vi "Read TemplatesFolder Key.vi"(8 "Error In":errorcluster) -> (0 "Error Out":errorcluster, 3 "Templates Folder Path":path)   [LabVIEW 2022 SP3]
doc: "This VI reads the path of the folder that stores the template VIs and CTLs from the \"TemplatesFolder\" value of the Windows Registry Key HKEY_CURRENT_USER\\Software\\NewViFromTemplate .\n\nIf the HKEY_CURRENT_USER\\Software\\NewViFromTemplate key doesn't exist, this VI creates it, and the \"TemplatesFolder\" value.\n\nIf the HKEY_CURRENT_USER\\Software\\NewViFromTemplate key exists, but the \"TemplatesFolder\" value doesn't, this VI creates the \"TemplatesFolder\" value.\n\nPetru, 07 November 2022"
uses:
  <vilib>/registry/registry.llb/Read Registry Value Simple STR.vi
  <vilib>/registry/registry.llb/Write Registry Value Simple STR.vi
panel:
  # "Development\nControls or indicators that are useful for development or testing, but which are not outputs of the VI."
  # "Input\nInputs to the VI"
  # "Output\nOutputs of the VI"
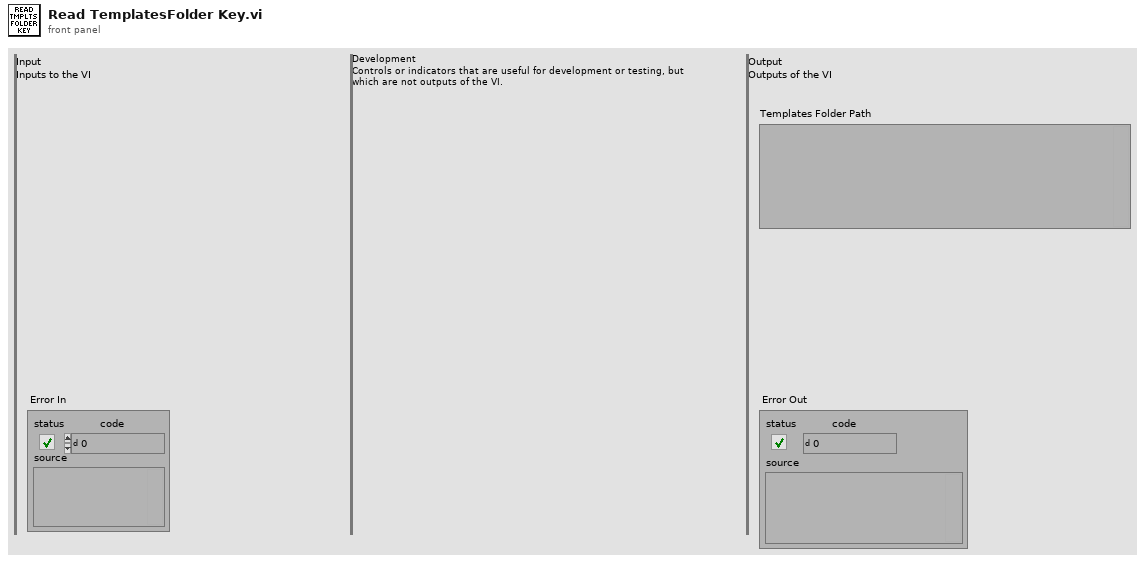
[diagram p1: front panel]
types:
  T1 = typedef "Registry RtKey.ctl" = enum32{"HKEY_CLASSES_ROOT", "HKEY_CURRENT_USER", "HKEY_LOCAL_MACHINE", "HKEY_USERS", "HKEY_PERFORMANCE_DATA", "HKEY_CURRENT_CONFIG", "HKEY_DYN_DATA"}
  T2 = typedef "Registry refnum.ctl" = refnum<k1>
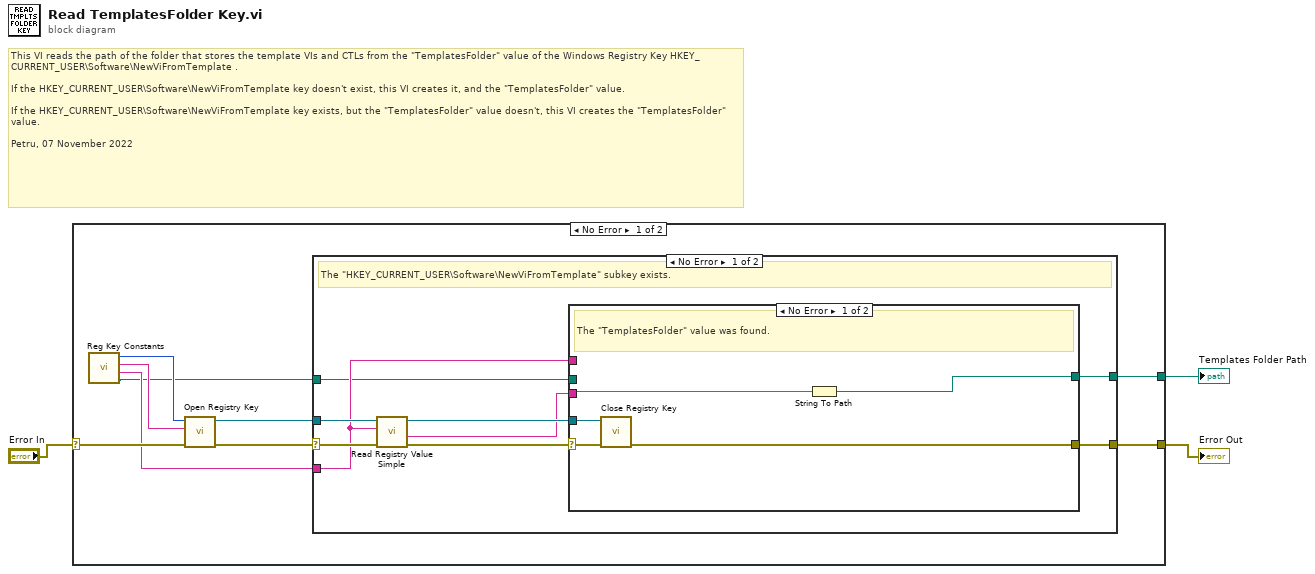
[diagram p0: block diagram]
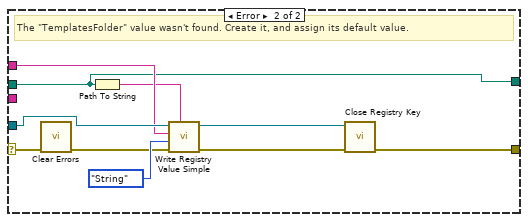
[diagram p2: hidden frame]
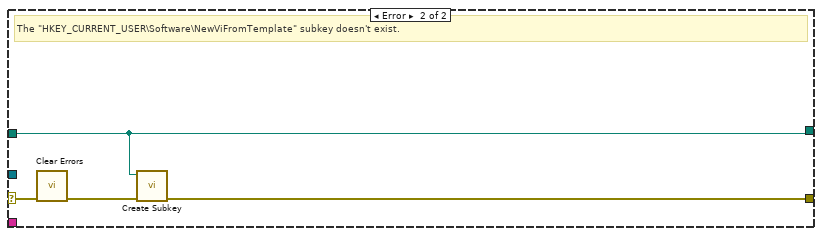
[diagram p3: hidden frame]
diagram:
  # "This VI reads the path of the folder that stores the template VIs and CTLs from the \"TemplatesFolder\" value of the Windows Registry Key HKEY_CURRENT_USER\\Software\\NewViFromTemplate .\n\nIf the HKEY_CURRENT_USER\\Software\\NewViFromTemplate key doesn't exist, this VI creates it, and the \"TemplatesFolder\" value.\n\nIf the HKEY_CURRENT_USER\\Software\\NewViFromTemplate key exists, but the \"TemplatesFolder\" value doesn't, this VI creates the \"TemplatesFolder\" value.\n\nPetru, 07 November 2022"
  n1 = case shown="No Error" "Error In" {
    selector: "Error In" -> [w12 w41]
    tunnel: [w10 w41] -> w2
    tunnel: [w8 _] -> w1
    frame No Error {
      n2 = call "Reg Key Constants.vi"() -> ("Default Templates Folder"=w4:path, "Name of TemplatesFolder Value"=w5:string, "Subkey Path"=w6:string, "Root Key"=w7:T1)  [unwired: 3 in, 1 out]
      n3 = call <vilib>:"Open Registry Key.vi"("error in (no error)"=w12, "subkey"=w6, "root key (HKEY_LOCAL_MACHINE)"=w7) -> ("error out"=w11:errorcluster, "refnum out"=w9:T2)  [unwired: 7 in]
      n4 = case shown="No Error" w11 {
        selector: w11 -> [w21 w40]
        tunnel: [w19 w39] -> w10
        tunnel: w9 -> [w17 _]
        tunnel: [w15 w38] -> w8
        tunnel: w5 -> [w14 _]
        tunnel: w4 -> [w13 w38]
        frame No Error {
          # "The \"HKEY_CURRENT_USER\\Software\\NewViFromTemplate\" subkey exists."
          n5 = call-poly <vilib>:"Read Registry Value Simple.vi"("error in (no error)"=w21, "value"=w14, "refnum"=w17) -> ("error out"=w20:errorcluster, "String/Binary data"=w16:string, "refnum out"=w18:T2)  [unwired: 3 in, 1 out]
          n6 = case shown="No Error" w20 {
            selector: w20 -> [w26 w35]
            tunnel: [w25 w31] -> w19
            tunnel: w18 -> [w24 w34]
            tunnel: w16 -> [w23 _]
            tunnel: [w22 w27] -> w15
            tunnel: w14 -> [_ w29]
            tunnel: w13 -> [_ w27]
            frame No Error {
              # "The \"TemplatesFolder\" value was found."
              n7 = call <vilib>:"Close Registry Key.vi"("error in (no error)"=w26, "refnum"=w24) -> ("error out"=w25:errorcluster)  [unwired: 5 in]
              n8 = String To Path(string=w23) -> (path=w22:path)
            }
            frame Error {
              # "The \"TemplatesFolder\" value wasn't found. Create it, and assign its default value."
              n9 = call <vilib>:"Clear Errors.vi"("error in (no error)"=w35) -> ("error out"=w33:errorcluster)  [unwired: 5 in, 1 out]
              n10 = Path To String(path=w27) -> (string=w28:string)
              n11 = call-poly <vilib>:"Write Registry Value Simple.vi"("String/Binary data"=w28, "error in (no error)"=w33, "simple data type"=enum16{"String", "Binary", "DWORD"}."String", "value"=w29, "refnum"=w34) -> ("error out"=w32:errorcluster, "refnum out"=w30:T2)  [unwired: 3 in]
              n12 = call <vilib>:"Close Registry Key.vi"("error in (no error)"=w32, "refnum"=w30) -> ("error out"=w31:errorcluster)  [unwired: 5 in]
            }
          }
        }
        frame Error {
          # "The \"HKEY_CURRENT_USER\\Software\\NewViFromTemplate\" subkey doesn't exist."
          n13 = call <vilib>:"Clear Errors.vi"("error in (no error)"=w40) -> ("error out"=w37:errorcluster)  [unwired: 5 in, 1 out]
          n14 = call "Create Subkey.vi"("Error In"=w37, "Default Templates Folder Path"=w38) -> ("Error Out"=w39:errorcluster)  [unwired: 8 in, 1 out]
        }
      }
    }
    frame Error {
    }
  }
  "Error Out" <- w2
  "Templates Folder Path" <- w1
